vi "TickCountDiff.vi"(9 "Count1":u32, 10 "Count2":u32) -> (2 "Diff (Count2-Count1)":u32)   [LabVIEW 2013]
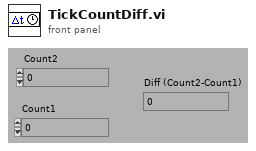
[diagram p1: front panel]
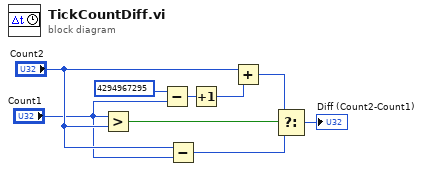
[diagram p0: block diagram]
diagram:
  n1 = Greater?(x="Count1", y="Count2") -> (0:w9:bool)
  n2 = Subtract(x=u32 4294967295 ("Count 1"), y="Count1") -> (x-y=w3:u32)
  n3 = Subtract(x="Count2", y="Count1") -> (x-y=w6:u32)
  n4 = Increment(x=w3) -> (x+1=w2:u32)
  n5 = Add(x="Count2", y=w2) -> (x+y=w1:u32)
  n6 = Select(t=w1, s=w9, f=w6) -> (s? t:f=→"Diff (Count2-Count1)":u32)
